vi "FPGA_AIReadAveraged.vi"(8 "error in (no error)":errorcluster, 10 "Channel":T1=enum."AI 1", 11 "AI Reference in":T2) -> (0 "error out":errorcluster, 2 "Averaged":i32, 3 "AI Reference out":T2)   [LabVIEW 2017]
uses:
  <vilib>/Rock Robotics/SystemInterfaces/AI/FPGA_AIDevRef.ctl
  <vilib>/Rock Robotics/SystemInterfaces/AI/FPGA_AIChannel.ctl
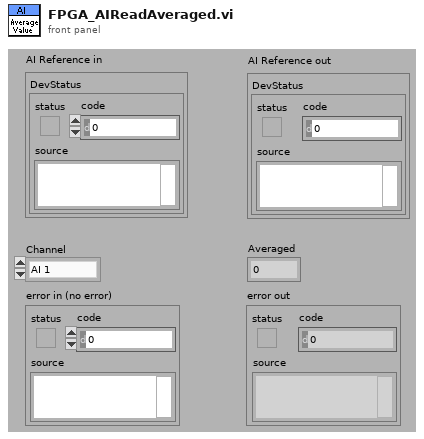
[diagram p1: front panel]
types:
  T1 = typedef "FPGA_AIChannel.ctl" = enum8{"AI 0", "AI 1", "AI 2", "AI 3", "AI MXP 0", "AI MXP 1", "AI MXP 2", "AI MXP 3", "Invalid"}
  T2 = typedef "FPGA_AIDevRef.ctl" = cluster{"DevStatus":errorcluster}
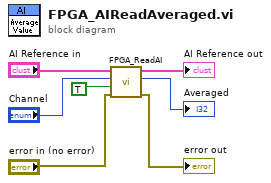
[diagram p0: block diagram]
diagram:
  n1 = call <vilib>:"FPGA_ReadAI.vi"("error in (no error)"="error in (no error)", "average?"=TRUE, "Channel"="Channel", "AI Reference"="AI Reference in") -> ("error out"=→"error out":errorcluster, "Value"=→"Averaged":i32, "AI Reference"=→"AI Reference out":T2)  [unwired: 5 out]
